vi "test Init Series Graph 1.vi"(11 "Test Case In":refnum<class "test Init Series Graph.lvclass">) -> (0 "error out":errorcluster, 3 "Test Case Out":refnum<class "test Init Series Graph.lvclass">)   [LabVIEW 2023, in "test Init Series Graph.lvclass"]
uses:
  test Init Series Graph.lvclass
  C:/Program Files/National Instruments/LabVIEW 2023/vi.lib/Astemes/LUnit/Test Case.lvclass
  source/Series Graph/Graph with Series View.lvclass
  <vilib>/Astemes/LUnit/Test Case.lvclass/Test Case.ctl
  <vilib>/Astemes/LUnit/Append Pass Result.vi
  <vilib>/Astemes/LUnit/Append Fail Result.vi
  <vilib>/Astemes/LUnit/Run In UI.vi
  <vilib>/Utility/error.llb/Clear Errors.vi
  test Init Series Graph.lvclass/test Init Series Graph.ctl
  <vilib>/Astemes/LUnit/Test Case.lvclass
panel:
  out "Z - Time Signal":dbl[](graph)
  out "Intensity Width Graph":cluster{"Array":dbl[], "Array":dbl[]}(graph)
  out "Signal Map":u16[][](graph)
  out "Intensity Height Graph":cluster{"Array":dbl[], "Array":dbl[]}(graph)
  in  "Image #":u16
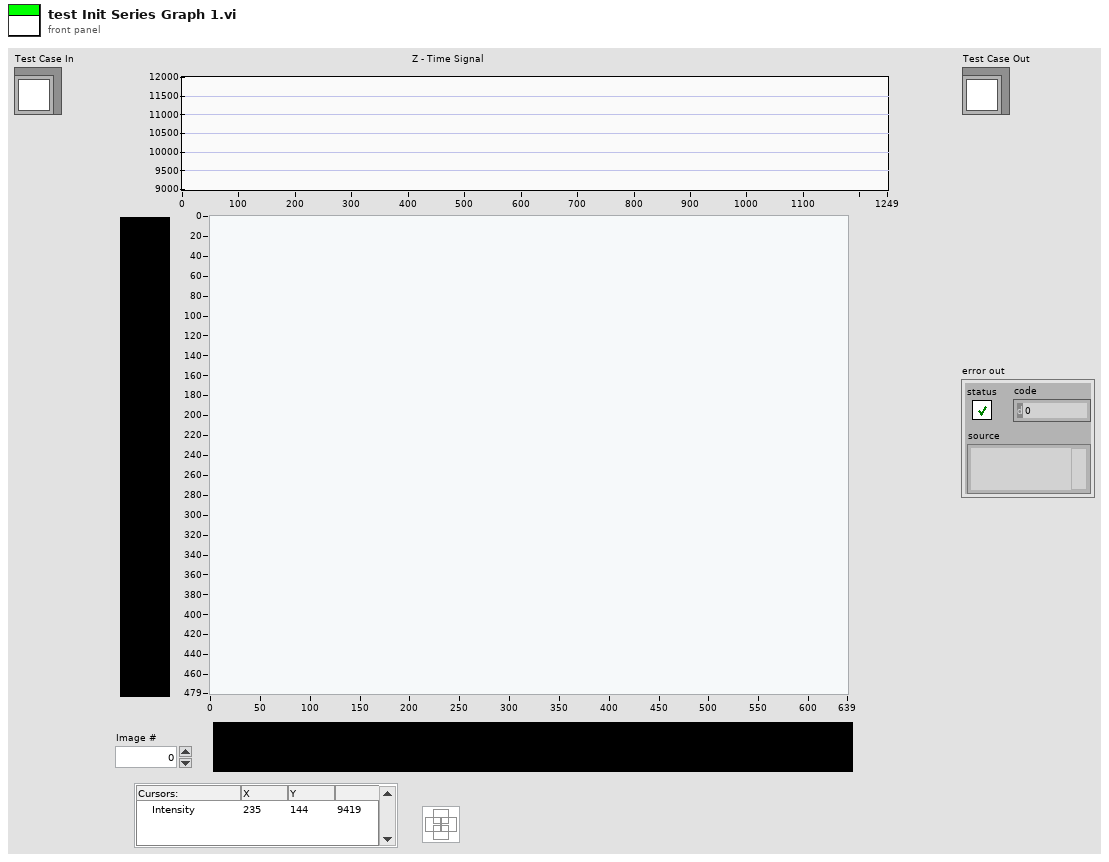
[diagram p1: front panel]
types:
  T1 = cluster{"Z-Graph":refnum<vi>, "IntGraph":refnum<vi>, "Y-Graph":refnum<vi>, "X-Graph":refnum<vi>}
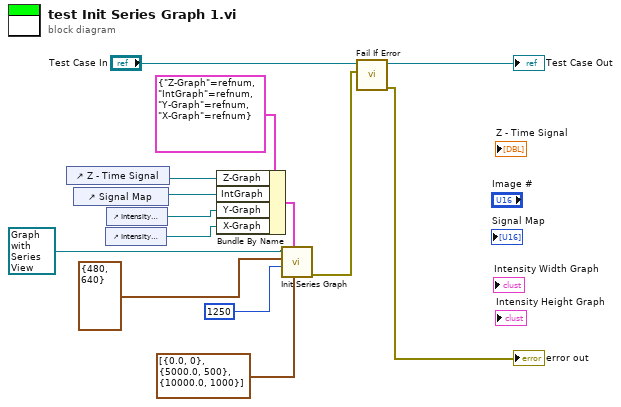
[diagram p0: block diagram]
diagram:
  n1 = control-ref of="Z - Time Signal"() -> (w8:refnum<vi>)
  n2 = control-ref of="Signal Map"() -> (w7:refnum<vi>)
  n3 = control-ref of="Intensity Width Graph"() -> (w5:refnum<vi>)
  n4 = control-ref of="Intensity Height Graph"() -> (w6:refnum<vi>)
  n5 = Bundle By Name(cluster=T1 {"Z-Graph"=refnum, "IntGraph"=refnum, "Y-Graph"=refnum, "X-Graph"=refnum} ("Graphs"), "Z-Graph"=w8, "IntGraph"=w7, "Y-Graph"=w6, "X-Graph"=w5) -> (w9:T1)
  n6 = call "Init Series Graph.vi"("Z Scale.Marker Values[]"=cluster{"Numeric":dbl, "Numeric":u32}[] [{"Numeric"=0.0, "Numeric"=0}, {"Numeric"=5000.0, "Numeric"=500}, {"Numeric"=10000.0, "Numeric"=1000}], "Graphs"=w9, "Shots"=u32 1250, "Image Size"=cluster{"Height":u32, "Width":u32} {"Height"=480, "Width"=640} ("Images Size"), "Series Graph in"=refnum<class "Graph with Series View.lvclass"> refnum) -> ("error out"=w1:errorcluster)  [unwired: 5 in, 1 out]
  n7 = call <vilib>:"Fail If Error.vi"("Assert error"=w1, "LUnit Test Case In"="Test Case In") -> ("error out"=→"error out":errorcluster, "LUnit Test Case Out"=→"Test Case Out":refnum<class "test Init Series Graph.lvclass">)  [unwired: 8 in]
